vi "general tcp data gatherer not complete.vi"() -> ()   [LabVIEW 2020]
uses:
  GUI_master/tcp new data cluster.ctl
  Device Driver/GUIDeviceInfo_TypDEf.ctl
  MySQL/Preset Query Enum.ctl
  TCP subscription info cluster.ctl
panel:
  in  "TCP subscriptions info":T1
  in  "stop":bool
  out "Requested values":string[](array[string])
  out "millisecond timer value":u32
  in  "Stop":bool
  in  "Expt name":string="Test"
  in  "GUIDeviceInfo":T2
  in  "tcp data event":refnum<user-event>
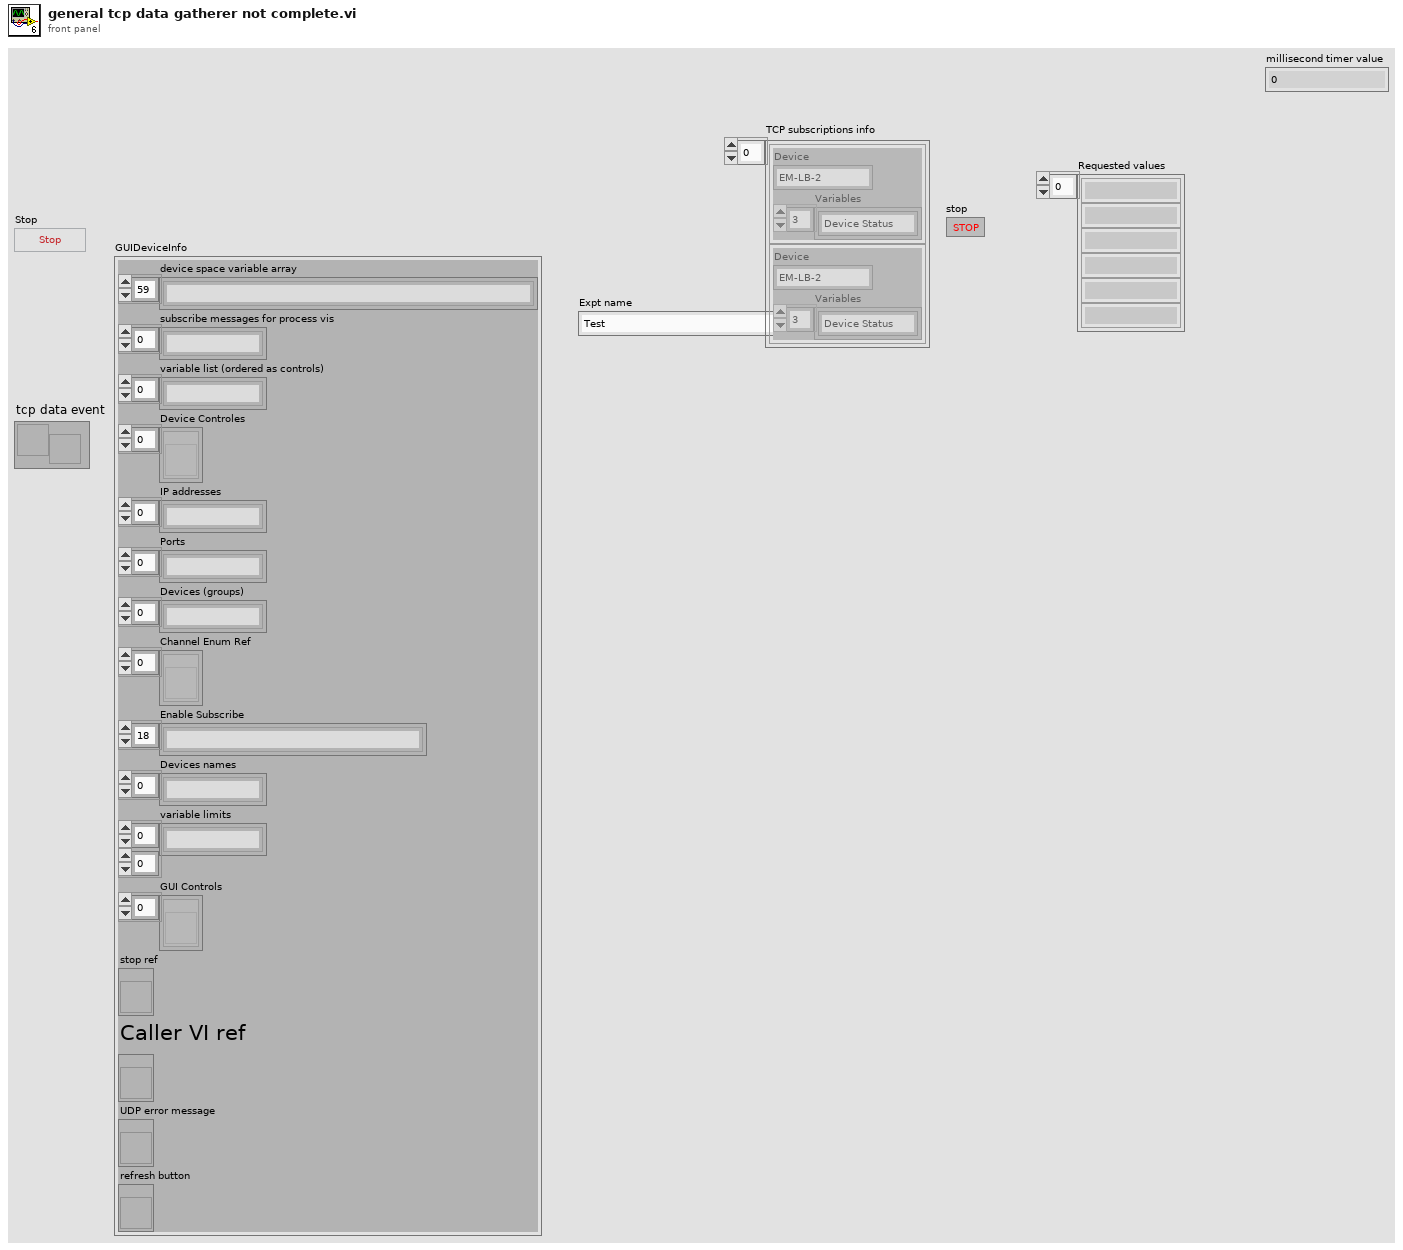
[diagram p1: front panel]
types:
  T1 = typedef "TCP subscription info cluster.ctl" = cluster{"Device":string, "Variables":string[]}[]
  T2 = typedef "GUIDeviceInfo_TypDEf.ctl" = cluster{"device space variable array":string[], "subscribe messages for process vis":string[], "variable list (ordered as controls)":string[], "Device Controles":refnum<vi>[], "IP addresses":string[], "Ports":string[], "Devices (groups)":string[], "Channel Enum Ref":refnum<vi>[], "Enable Subscribe":string[], "Devices names":string[], "variable limits":string[][], "GUI Controls ":refnum<vi>[], "stop ref":refnum<vi>, "Caller VI ref":refnum<vi>, "UDP error message":refnum<vi>, "refresh button":refnum<vi>}
  T3 = typedef "Preset Query Enum.ctl" = enum16{"Get Locations", "Get all IPs and MACs", "Get classes", "Get expt variables to set at scanstart for particular device", "Get expt devices and variables with start values", "Get expt devices and variables (with data to get)", "Get expt devices with data to get", "Get Expt devices and GUIs", "Get all devices basic properties", "Get Virtual Devices Core Info", "Get Expt names", "Get experiment basic properties", "Get experiment alarm variables", "Get MC Ports", "Get device network comm port", "Get devicetype lvclass path", "Get basic device properties", "Get Init Order", "Get all setable variables of a device", "Get device variable aliases", "Get force values of all settable variables", "Get all variables of a devicetype", "Get all variables of a device", "Get plotter details", "Get Saved Scans", "Get Scan Info", "GetGeneralGUIs", "Get expt for plotter", "Get plotter IDs from expt", "Get all devices", "Get all Virtual Devices", "Get all aliases", "Get variable and device info for Virtual Device", "GetItemLocatorIP", "Get IPs for GUIs", "Get DeviceType from Device", "GetLocalPortRange", "GetDevicePresetVariables", "Get Device Configuration", "GetAllPresetNames", "GetAllConfigurationNames", "GetPresetDeviceNames", "GetDeviceAliases", "GetDevicesOfClass"}
  T4 = typedef "QueueCluster.ctl" = cluster{"UDP":refnum<queue>, "Data":refnum<queue>, "Stop":refnum<queue>, "Control":refnum<queue>, "tcp data event":refnum<user-event>, "Event Registration Refnum":refnum<event-registration>}
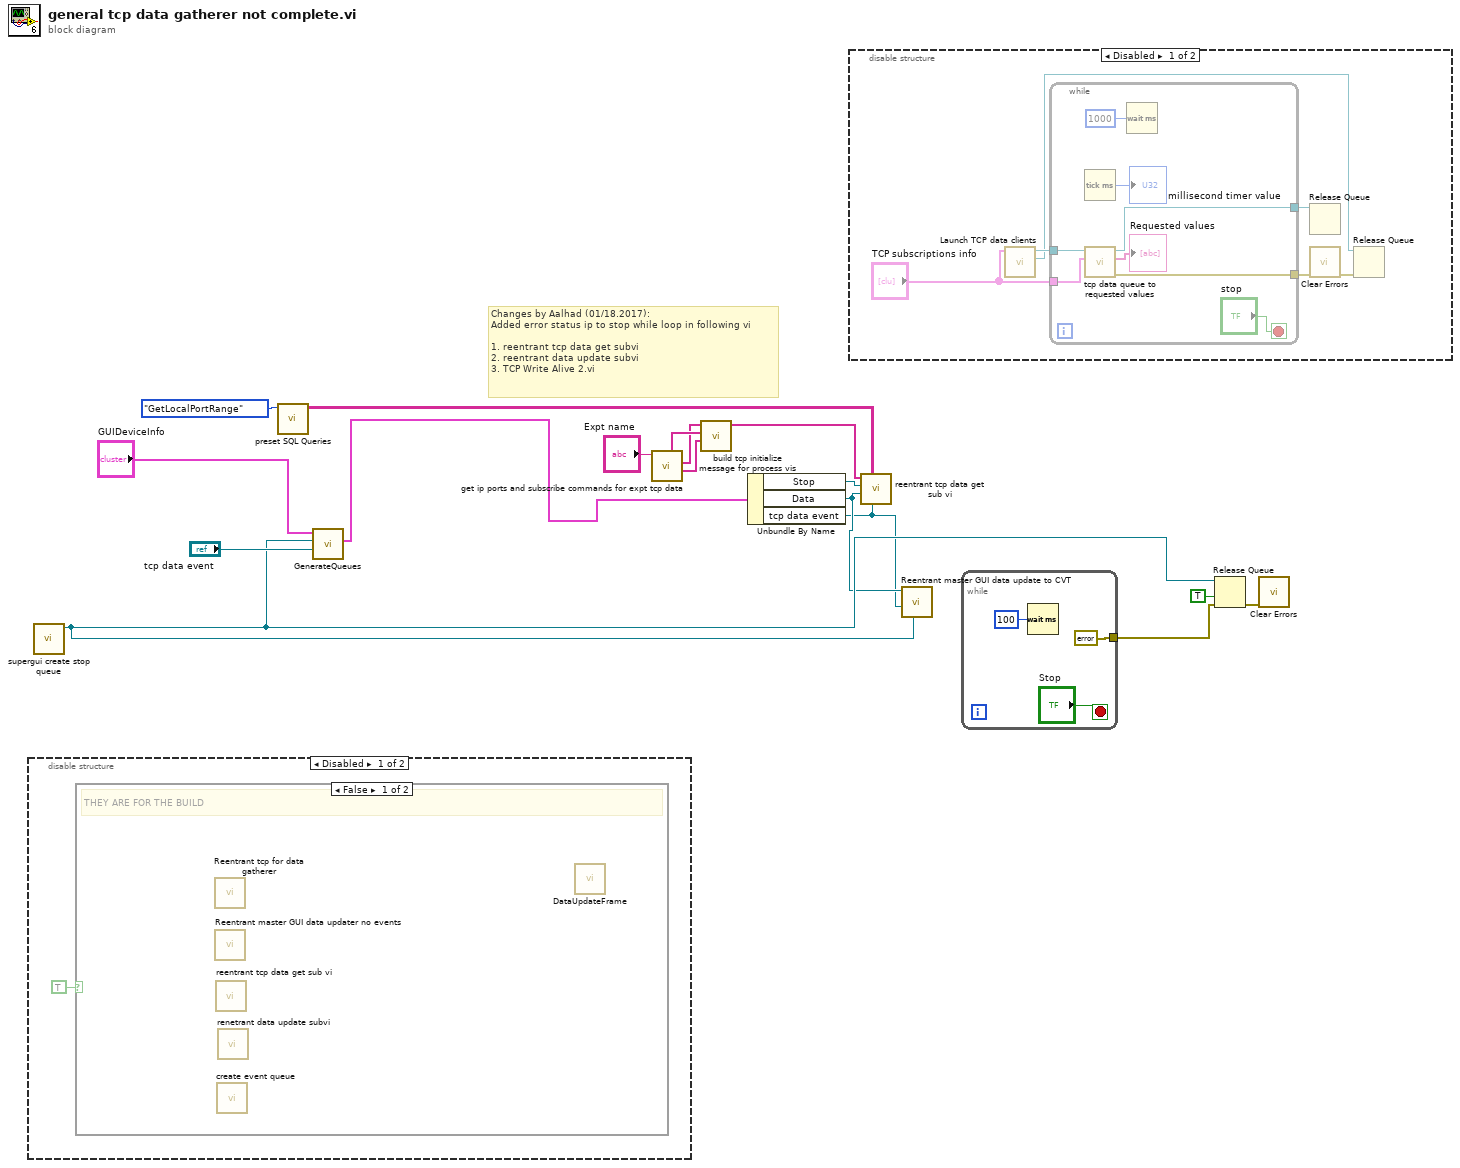
[diagram p0: block diagram]
diagram:
  # "Changes by Aalhad (01/18.2017):\nAdded error status ip to stop while loop in following vi\n\n1. reentrant tcp data get subvi\n2. reentrant data update subvi\n3. TCP Write Alive 2.vi"
  n1 = disable-structure shown="Disabled" {
    frame Disabled {
      n2 = case shown="False" TRUE {
        frame False {
          # "THEY ARE FOR THE BUILD"
          n3 = call "Reentrant tcp for data gatherer.vi"() -> ()  [unwired: 1 in]
          n4 = call "Reentrant master GUI data updater no events.vi"() -> ()  [unwired: 12 in]
          n5 = call "reentrant tcp data get sub vi.vi"() -> ()  [unwired: 11 in, 1 out]
          n6 = call "create event queue.vi"() -> ()  [unwired: 10 in, 2 out]
          n7 = call "renetrant data update subvi.vi"() -> ()  [unwired: 8 in]
          n8 = call "DataUpdateFrame.vi"() -> ()  [unwired: 11 in, 1 out]
        }
        frame True {
        }
      }
    }
    frame Enabled {
    }
  }
  n9 = call "supergui create stop queue.vi"() -> ("STOP Queue out"=w3:refnum<queue>)  [unwired: 11 in]
  n10 = call "preset SQL Queries.vi"("Preset Query"=Preset_Query_Enum."GetLocalPortRange") -> ("data"=w14:string[][])  [unwired: 8 in, 2 out]
  n11 = call "GenerateQueues.vi"("User Event in"="tcp data event", "STOP Queue in"=w3, "GUIDeviceInfo"="GUIDeviceInfo") -> ("Queue Cluster"=w10:T4)  [unwired: 4 in, 4 out]
  n12 = call "get ip ports and subscribe commands for expt tcp data.vi"("Device/Devicetype name\n/Plotter.id/#"="Expt name") -> ("IP Addresses"=w7:string[], "Subscribe commands"=w6:string[], "Ports"=w8:string[])  [unwired: 6 in, 2 out]
  n13 = call "build tcp initialize message for process vis.vi"("IP Addresses"=w7, "Ports"=w8, "Subscribe commands"=w6) -> ("subscribe messages\nfor process vis"=w5:string[])  [unwired: 8 in]
  n14 = Unbundle By Name(w10) -> ("Stop"=w13:refnum<queue>, "Data"=w2:refnum<queue>, "tcp data event"=w1:refnum<user-event>)
  n15 = disable-structure shown="Disabled" {
    frame Disabled {
      n16 = call "Launch TCP data clients.vi"("TCP subscriptions info"="TCP subscriptions info") -> ("StopQueue"=w22:refnum<queue>, "DataQueue"=w24:refnum<queue>)  [unwired: 8 in, 1 out]
      n17 = while {
        tunnel: w24 -> [w31]
        tunnel: [w30] -> w23
        tunnel: [w29] -> w21
        tunnel: "TCP subscriptions info" -> [w26]
        stop <- "stop" stop-if-true
        n18 = Tick Count (ms)() -> (millisecond timer value=→"millisecond timer value":u32)
        n19 = call "tcp data queue to requested values.vi"("TCP subscriptions info"=w26, "Queue in"=w31) -> ("error out"=w29:errorcluster, "Array"=→"Requested values":string[], "Queue out"=w30:refnum<queue>)  [unwired: 7 in]
        n20 = Wait (ms)(milliseconds to wait=u32 1000) -> ()  [unwired: 1 out]
      }
      n21 = Release Queue(queue=w23) -> ()  [unwired: 2 in, 3 out]
      n22 = call <vilib>:"Clear Errors.vi"("error in (no error)"=w21) -> ("error out"=w20:errorcluster)  [unwired: 5 in, 1 out]
      n23 = Release Queue(queue=w22, error in (no error)=w20) -> ()  [unwired: 1 in, 3 out]
    }
    frame Enabled {
    }
  }
  n24 = call "reentrant tcp data get sub vi.vi"("tcp data event"=w1, "Ports"=w14, "tcpDataqueue"=w2, "Stopqueue"=w13, "subscribe messages for process vis"=w5) -> ()  [unwired: 6 in, 1 out]
  n25 = call "Reentrant master GUI data update to CVT.vi"("Stopqueue"=w3, "tcp data event"=w1, "tcpDataqueue"=w2) -> ()  [unwired: 9 in]
  n26 = while {
    tunnel: [errorcluster {"status"=FALSE, "code"=0, "source"=""} ("error out")] -> w4
    stop <- "Stop" stop-if-true
    n27 = Wait (ms)(milliseconds to wait=u32 100) -> ()  [unwired: 1 out]
  }
  n28 = Release Queue(queue=w3, force destroy? (F)=TRUE, error in (no error)=w4) -> (error out=w11:errorcluster)  [unwired: 2 out]
  n29 = call <vilib>:"Clear Errors.vi"("error in (no error)"=w11) -> ()  [unwired: 5 in, 2 out]
